vi "ScpChTrIsAvailable.vi"(8 "error in (no error)":errorcluster, 10 "wCh in":u16, 11 "hDevice in":u32) -> (0 "error out":errorcluster, 1 "bIsAvailable":bool, 2 "wCh out":u16, 3 "hDevice out":u32)   [LabVIEW 2018, in "LibTiePie.lvlib"]
uses:
  LibTiePie.lvlib
  LabViewHS4/libtiepie.dll
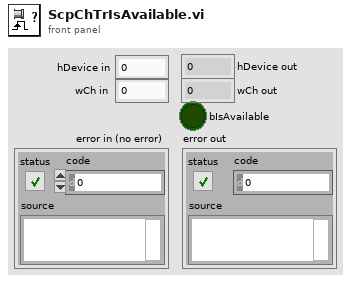
[diagram p1: front panel]
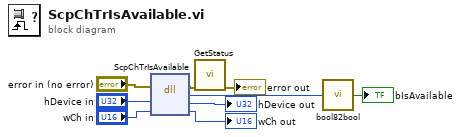
[diagram p0: block diagram]
diagram:
  n1 = dll-call lib="C:/Users/cwaha/Documents/LabViewHS4/libtiepie.dll" fn="ScpChTrIsAvailable"(error in="error in (no error)", "hDevice"="hDevice in", "wCh"="wCh in") -> (error out=w9:errorcluster, "bAvailable"=w7:u8, "hDevice"=→"hDevice out":u32, "wCh"=→"wCh out":u16)  [unwired: 2 in, 1 out]
  n2 = call "GetStatus.vi"("error in (no error)"=w9) -> ("error out"=→"error out":errorcluster)  [unwired: 10 in]
  n3 = call "bool82bool.vi"("bool8 in"=w7) -> ("bool out"=→"bIsAvailable":bool)
